vi "Configure Ports.vi"(8 "error in (no error)":errorcluster, 10 "Array of line":T1[](array[typedef]), 11 "National Instrument USB-6501 in":refnum<class "National Instrument USB-6501.lvclass">) -> (0 "error out":errorcluster, 3 "National Instrument USB-6501 out":refnum<class "National Instrument USB-6501.lvclass">)   [LabVIEW 2016, in "Generic Data Acquisition.lvlib" / "National Instrument USB-6501.lvlib" / "National Instrument USB-6501.lvclass"]
uses:
  National Instrument USB-6501.lvclass
  Controls/Data Acquisition Channel Settings.ctl
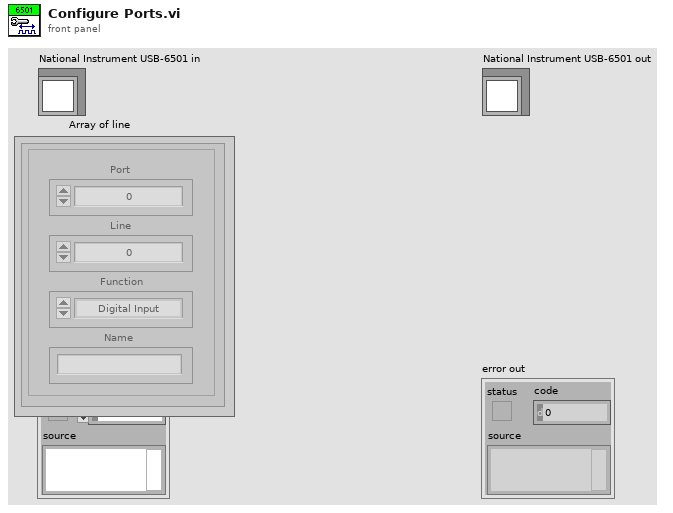
[diagram p1: front panel]
types:
  T1 = typedef "Data Acquisition Channel Settings.ctl" = cluster{"Function":enum16{"Digital Input", "Digital Output"}, "Port":i8, "Line":i8, "Name":string}
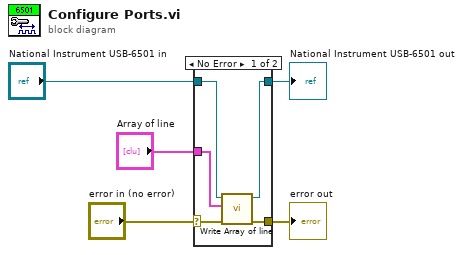
[diagram p0: block diagram]
diagram:
  n1 = case shown="No Error" "error in (no error)" {
    selector: "error in (no error)" -> [w8 w12]
    tunnel: [w7 w12] -> w4
    tunnel: [w9 w11] -> w2
    tunnel: "National Instrument USB-6501 in" -> [w10 w11]
    tunnel: "Array of line" -> [w6 _]
    frame No Error {
      n2 = call-dynamic "Write Array of line.vi"("error in (no error)"=w8, "Array of line"=w6, "National Instrument USB-6501 in"=w10) -> ("error out"=w7:errorcluster, "National Instrument USB-6501 out"=w9:refnum<class "National Instrument USB-6501.lvclass">)  [unwired: 7 in]
    }
    frame Error {
    }
  }
  "error out" <- w4
  "National Instrument USB-6501 out" <- w2
